vi "Unregister Event.vi"(8 "Error In":errorcluster, 9 "Registrant Address":refnum<class "Message Enqueuer.lvclass">, 10 "Event":refnum<class "Event.lvclass">, 11 "Controller Actor In":refnum<class "Controller Actor.lvclass">) -> (0 "Error Out":errorcluster, 3 "Controller Actor Out":refnum<class "Controller Actor.lvclass">)   [LabVIEW 2017, in "Event Actors.lvlib" / "Controller Actor.lvclass"]
doc: "This method unregisters a specific Actors Enqueuer from specific Event he is listening to, in this Event Source Actor."
uses:
  Controller Actor.lvclass
  <vilib>/ActorFramework/Message Enqueuer/Message Enqueuer.lvclass
  Event/Event.lvclass
  Controller Actor.lvclass/Controller Actor.ctl
  Event/Event.lvclass/Event.ctl
  <resource>/AFDebug/Generate Trace.vi
  <resource>/AFDebug/TDM Registry.vi
  <resource>/AFDebug/Localized Strings.vi
  <resource>/AFDebug/Actor Registry.vi
  <resource>/AFDebug/Get Clone Name.vi
  <resource>/AFDebug/AF Debug.lvlib
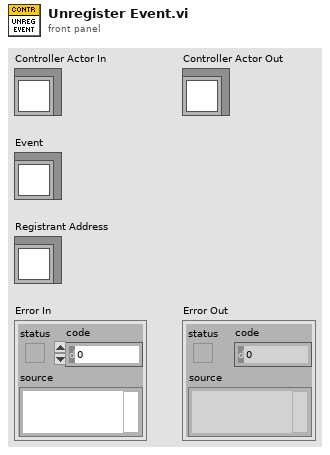
[diagram p1: front panel]
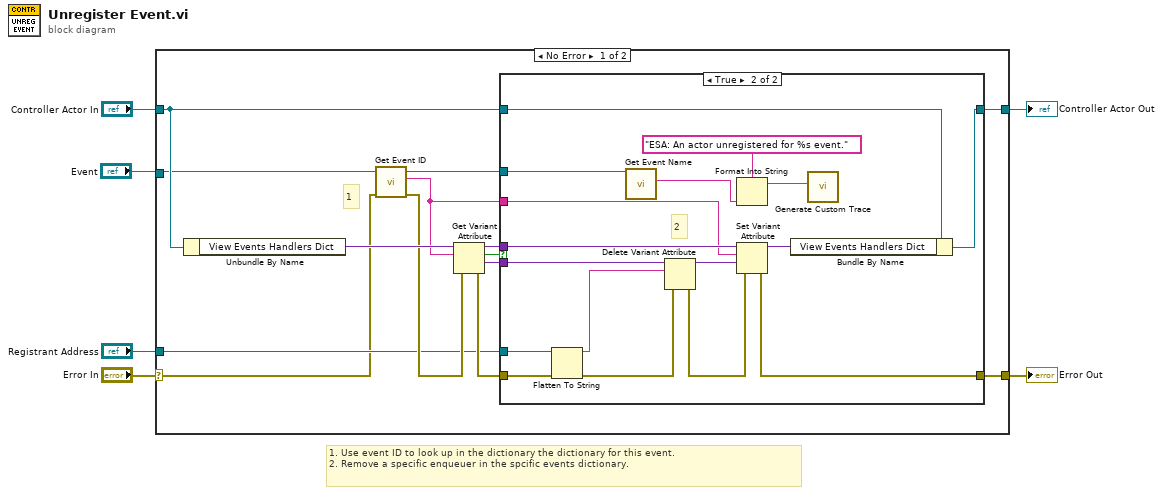
[diagram p0: block diagram]
diagram:
  # "1. Use event ID to look up in the dictionary the dictionary for this event.\n2. Remove a specific enqueuer in the spcific events dictionary."
  n1 = case shown="No Error" "Error In" {
    selector: "Error In" -> [w7 w41]
    tunnel: "Registrant Address" -> [w8 _]
    tunnel: [w20 w41] -> w5
    tunnel: "Event" -> [w12 _]
    tunnel: "Controller Actor In" -> [w13 w40]
    tunnel: [w14 w40] -> w1
    frame No Error {
      # "1"
      n2 = Unbundle By Name(w13) -> ("View Events Handlers Dict"=w19:variant)
      n3 = call-dynamic "Get Event ID.vi"("error in (no error)"=w7, "Event in"=w12) -> ("error out"=w9:errorcluster, "Event ID"=w10:string, "Event out"=w11:refnum<class "Event.lvclass">)  [unwired: 7 in]
      n4 = Get Variant Attribute(Variant=w19, name=w10, error in=w9) -> (duplicate Variant=w15:variant, found=w16:bool, value=w17:variant, error out=w18:errorcluster)  [unwired: 1 in]
      n5 = case shown="True" w16 {
        tunnel: w17 -> [_ w39]
        tunnel: w8 -> [_ w23]
        tunnel: w18 -> [w22 w26]
        tunnel: [w22 w35] -> w20
        tunnel: w15 -> [_ w38]
        tunnel: w10 -> [_ w29]
        tunnel: w13 -> [w21 w34]
        tunnel: [w21 w32] -> w14
        tunnel: w11 -> [_ w28]
        frame False {
        }
        frame True {
          # "2"
          n6 = Flatten To String(anything=w23, error in (no error)=w26) -> (data string=w24:string, error out=w25:errorcluster)  [unwired: 2 in, 1 out]
          n7 = call "Get Event Name.vi"("Event In"=w28) -> ("Name"=w27:string)  [unwired: 9 in, 1 out]
          n8 = Delete Variant Attribute(4:w25, 6:w24, 7:w39) -> (0:w36:errorcluster, 3:w37:variant)  [unwired: 1 out]
          n9 = Format Into String(format string="ESA: An actor unregistered for %s event." ("Custom Action"), w27) -> (resulting string=w30:string)  [unwired: 2 in, 1 out]
          n10 = Set Variant Attribute(Variant=w38, name=w29, value=w37, error in=w36) -> (Variant out=w33:variant, error out=w35:errorcluster)  [unwired: 1 out]
          n11 = Bundle By Name(cluster=w34, "View Events Handlers Dict"=w33) -> (w32:refnum<class "Controller Actor.lvclass">)
          n12 = call <resource>:"Generate Custom Trace.vi"("Custom Action"=w30) -> ()  [unwired: 11 in]
        }
      }
    }
    frame Error {
    }
  }
  "Error Out" <- w5
  "Controller Actor Out" <- w1
